vi "ni_monoDrive.vi"() -> ()   [LabVIEW 2018]
uses:
  f4205ffc-a547-4453-97f1-55d6d4306e88.vi
panel:
  out "error out":errorcluster
  out "sensor error":errorcluster
  in  "Tab Control":enum32{"Vehicle", "Environment"}(tab)
  out "Sensor Config":string
  in  "Sensor Configuration":path
  in  "Simulator Configuration":path
  out "Simulator Config":string
  in  "Python Module Path":path
  in  "Steering Angle":dbl(knob) scale=-1.0..1.0
  out "Waveform Chart":dbl(graph)
  out "Speed":dbl(knob) scale=0.0..200.0
  in  "stop":bool
  in  "Throttle":dbl(slide) scale=-1.0..1.0
  out "camera_out 2":picture
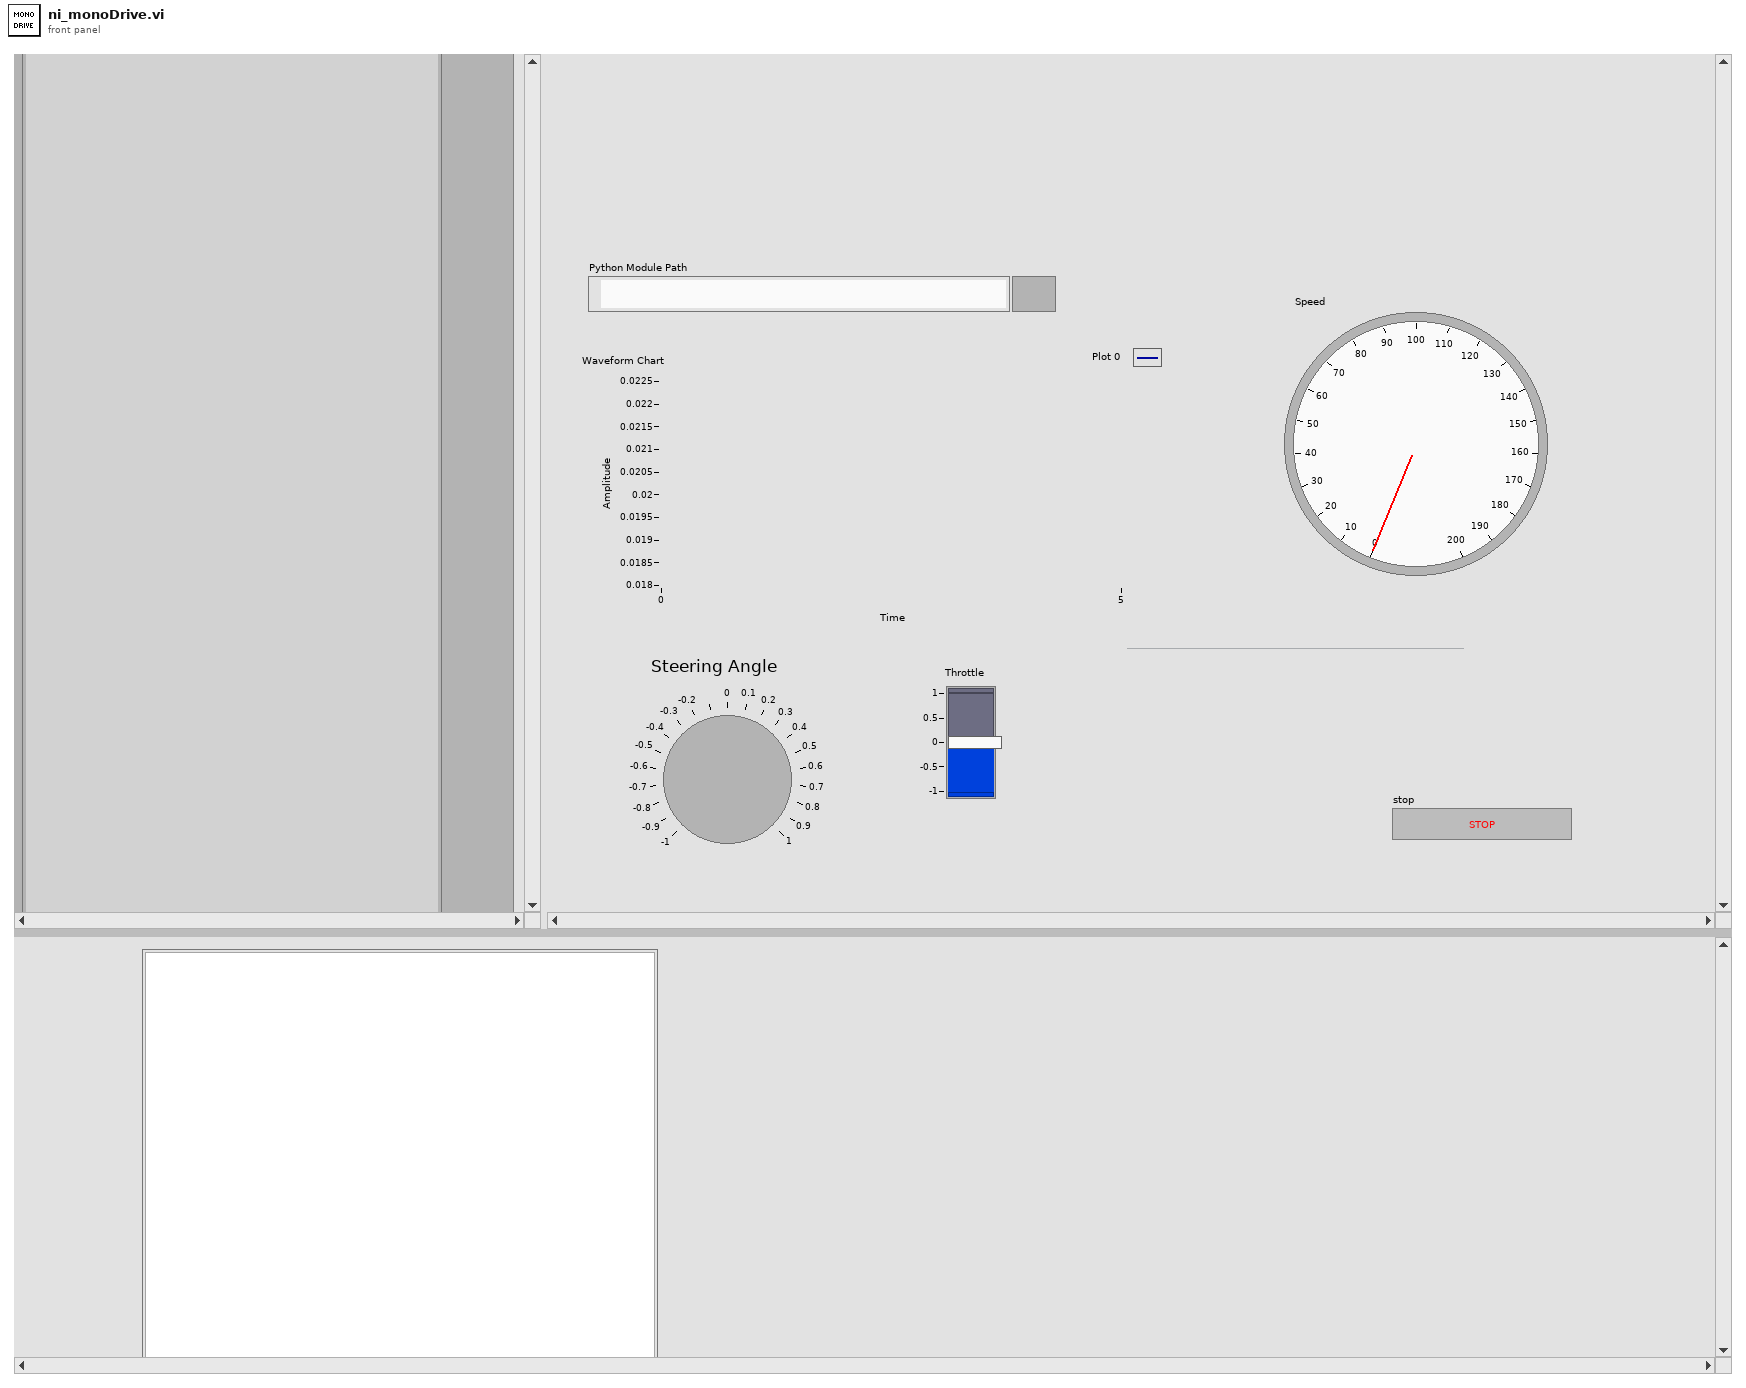
[diagram p1: front panel]
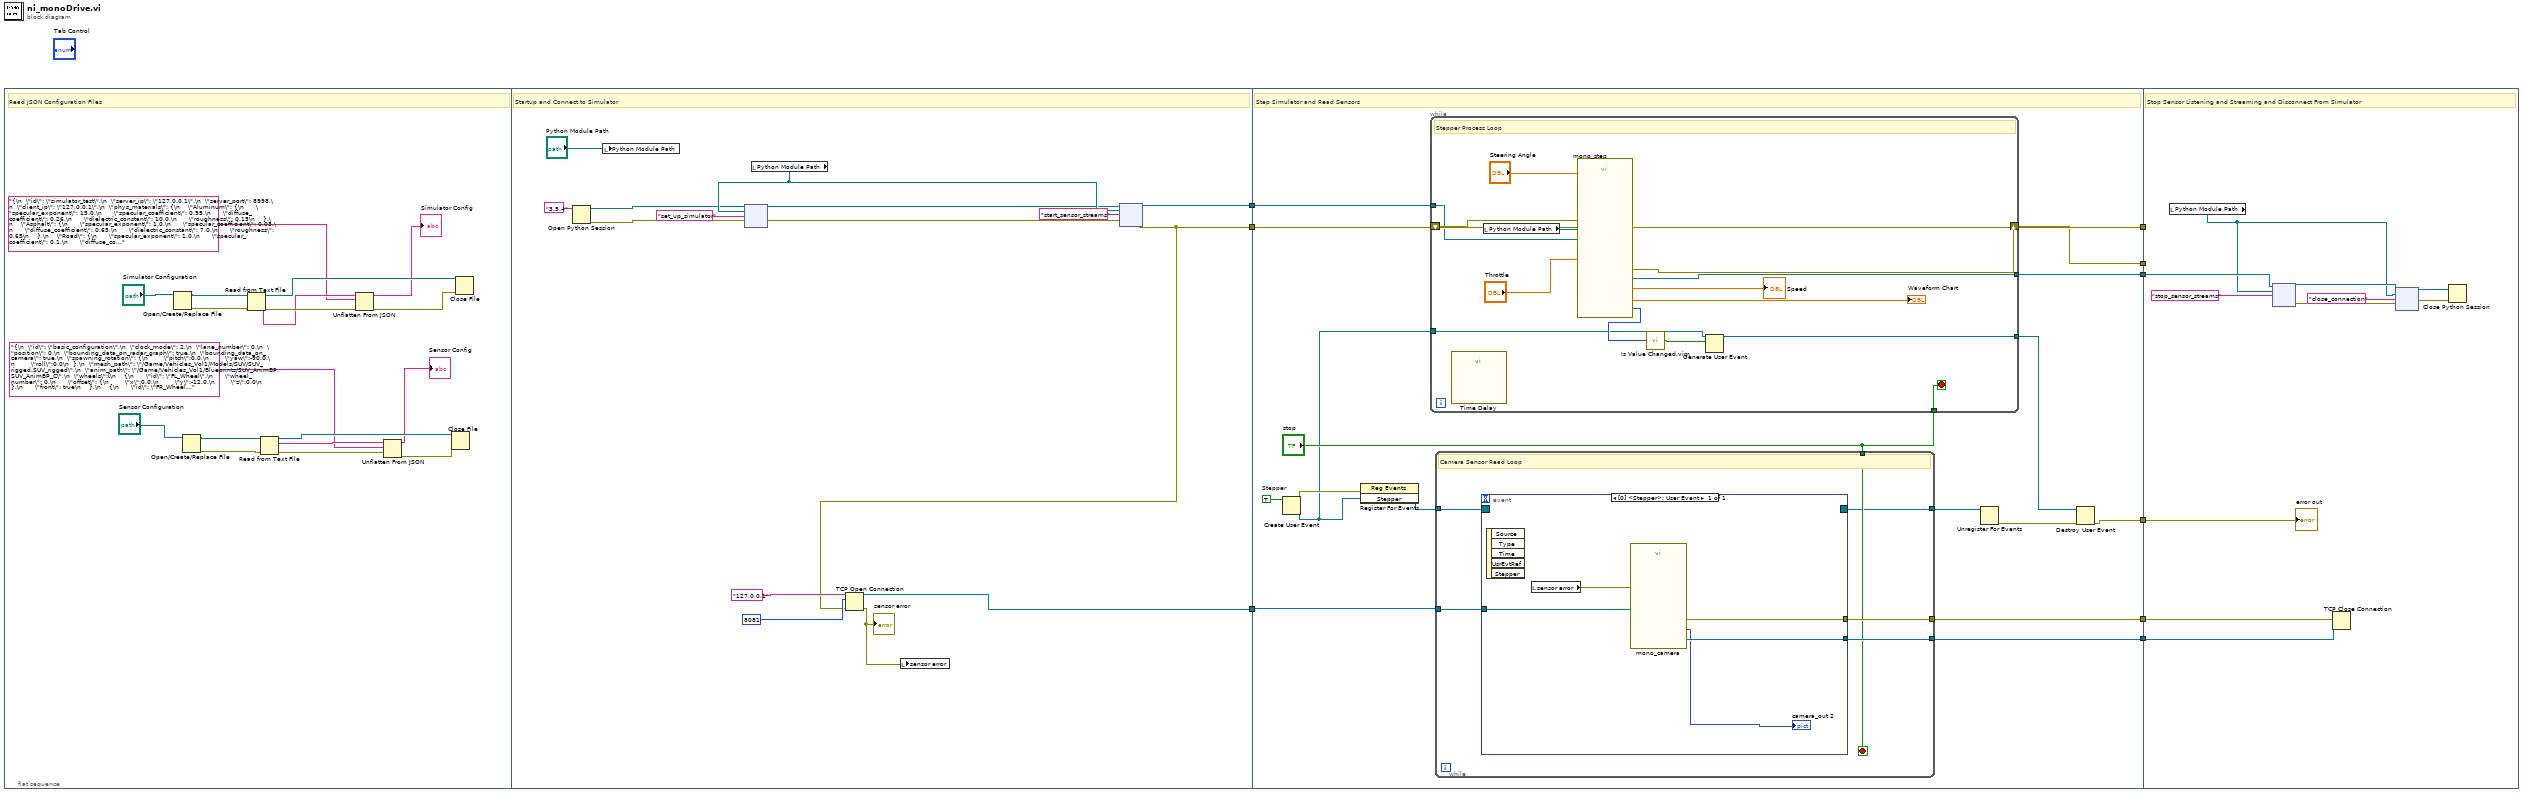
[diagram p0: block diagram]
diagram:
  n1 = flat-sequence {
    tunnel: [w28] -> w9
    tunnel: [w30] -> w4
    tunnel: [w29] -> w3
    tunnel: w9 -> [w58]
    tunnel: [w58] -> w8
    tunnel: [w57] -> w7
    tunnel: [w56] -> w6
    tunnel: [w55] -> w5
    tunnel: w4 -> [w54]
    tunnel: w3 -> [w53]
    tunnel: [w52] -> w2
    tunnel: [w47] -> w1
    tunnel: w8 -> [_]
    tunnel: w7 -> [_]
    tunnel: w6 -> [w88]
    tunnel: w5 -> [w87]
    tunnel: w2 -> [w86]
    tunnel: w1 -> [w84]
    frame #0 {
      # "Read JSON Configuration Files"
      n2 = Open/Create/Replace File(file path (use dialog)="Simulator Configuration") -> (refnum out=w17:refnum<file>, error out=w15:errorcluster)  [unwired: 5 in, 1 out]
      n3 = Open/Create/Replace File(file path (use dialog)="Sensor Configuration") -> (refnum out=w26:refnum<file>, error out=w24:errorcluster)  [unwired: 5 in, 1 out]
      n4 = Read from Text File(file (use dialog)=w17, error in=w15) -> (refnum out=w16:refnum<file>, text=w12:string, error out=w14:errorcluster)  [unwired: 2 in, 1 out]
      n5 = Read from Text File(file (use dialog)=w26, error in=w24) -> (refnum out=w25:refnum<file>, text=w21:string, error out=w23:errorcluster)  [unwired: 2 in, 1 out]
      n6 = Unflatten From JSON(JSON string=w12, type and defaults="{\n  \"id\": \"simulator_test\",\n  \"server_ip\": \"127.0.0.1\",\n  \"server_port\": 8998,\n  \"client_ip\": \"127.0.0.1\",\n  \"phys_materials\": {\n    \"Aluminum\": {\n      \"specular_exponent\": 15.0,\n      \"specular_coefficient\": 0.95,\n      \"diffuse_coefficient\": 0.26,\n      \"dielectric_constant\": 10.0,\n      \"roughness\": 0.15\n    },\n    \"Asphalt\": {\n      \"specular_exponent\": 1.0,\n      \"specular_coefficient\": 0.03,\n      \"diffuse_coefficient\": 0.65,\n      \"dielectric_constant\": 7.0,\n      \"roughness\": 0.65\n    },\n    \"Road\": {\n      \"specular_exponent\": 1.0,\n      \"specular_coefficient\": 0.1,\n      \"diffuse_coefficient\": 0.65,\n      \"dielectric_constant\": 7.0,\n      \"roughness\": 0.65\n    },\n    \"Concrete\": {\n      \"specular_exponent\": 0.0,\n      \"specular_coefficient\": 0.1,\n      \"diffuse_coefficient\": 0.65,\n      \"dielectric_constant\": 7.0,\n      \"roughness\": 0.0\n    },\n    \"Glass\": {\n      \"specular_exponent\": 80.0,\n      \"specular_coefficient\": 0.80,\n      \"diffuse_coefficient\": 0.15,\n      \"dielectric_constant\": 4.0,\n      \"roughness\": 0.10\n    },\n    \"LandScape\": {\n      \"specular_exponent\": 10.0,\n      \"specular_coefficient\": 0.50,\n      \"diffuse_coefficient\": 0.50,\n      \"dielectric_constant\": 10.0,\n      \"roughness\": 0.60\n    },\n    \"Plastic\": {\n      \"specular_exponent\": 25.0,\n      \"specular_coefficient\": 0.40,\n      \"diffuse_coefficient\": 0.60,\n      \"dielectric_constant\": 2.8,\n      \"roughness\": 0.09\n    },\n    \"Steel\": {\n      \"specular_exponent\": 26.0,\n      \"specular_coefficient\": 1.0,\n      \"diffuse_coefficient\": 0.33,\n      \"dielectric_constant\": 0.0,\n      \"roughness\": 0.23\n    },\n    \"Tree\": {\n      \"specular_exponent\": 10.0,\n      \"specular_coefficient\": 0.05,\n      \"diffuse_coefficient\": 0.97,\n      \"dielectric_constant\": 10.0,\n      \"roughness\": 0.60\n    },\n    \"Wheel\": {\n      \"specular_exponent\": 92.0,\n      \"specular_coefficient\": 0.95,\n      \"diffuse_coefficient\": 0.06,\n      \"dielectric_constant\": 10.0,\n      \"roughness\": 0.15\n    },\n    \"Tire\": {\n      \"specular_exponent\": 25.0,\n      \"specular_coefficient\": 0.40,\n      \"diffuse_coefficient\": 0.60,\n      \"dielectric_constant\": 2.8,\n      \"roughness\": 0.15\n    }\n  },\n  \"traffic_configuration\": {\n    \"max_vehicles\": 40,\n    \"spawn_rate\": 0.25\n  },\n  \"client_settings\": {\n    \"map\": {\n      \"gis_anchor\": { \"x\": 0, \"y\": 0, \"z\": 0},\n      \"point_delta\": 100.0\n    },\n    \"gui\":{\n      \"fps\": 1.0\n    },\n    \"logger\": {\n      \"sensor\": \"debug\",\n      \"network\": \"debug\",\n      \"control\": \"debug\",\n      \"scenario\": \"debug\",\n      \"simulator\": \"debug\",\n      \"vehicle\": \"debug\"\n    }\n  }\n}\n" ("function name"), error in (no error)=w14) -> (value=→"Simulator Config":string, error out=w13:errorcluster)  [unwired: 4 in]
      n7 = Unflatten From JSON(JSON string=w21, type and defaults="{\n  \"id\": \"basic_configuration\",\n  \"clock_mode\": 2,\n  \"lane_number\": 0,\n  \"position\": 0,\n  \"bounding_data_on_radar_graph\": true,\n  \"bounding_data_on_camera\": true,\n  \"spawning_rotation\": {\n        \"pitch\":0.0,\n        \"yaw\":-90.0,\n        \"roll\":0.0\n  },\n  \"mesh_path\": \"/Game/Vehicles_Vol1/Models/SUV/SUV_rigged.SUV_rigged\",\n  \"anim_path\": \"/Game/Vehicles_Vol1/Blueprints/SUV_AnimBP.SUV_AnimBP_C\",\n  \"wheels\":[\n    {\n      \"id\": \"FL_Wheel\",\n      \"wheel_number\": 0,\n      \"offset\": {\n        \"x\":0.0,\n        \"y\":-12.0,\n        \"z\":0.0\n      },\n      \"front\": true\n    },\n    {\n      \"id\": \"FR_Wheel\",\n      \"wheel_number\": 1,\n      \"offset\": {\n        \"x\":0.0,\n        \"y\":12.0,\n        \"z\":0.0\n      },\n      \"front\": true\n    },\n    {\n      \"id\": \"BL_Wheel\",\n      \"wheel_number\": 2,\n      \"offset\": {\n        \"x\":0.0,\n        \"y\":-12.0,\n        \"z\":0.0\n      },\n      \"front\": false\n    },\n    {\n      \"id\": \"BR_Wheel\",\n      \"wheel_number\": 3,\n      \"offset\": {\n        \"x\":0.0,\n        \"y\":12.0,\n        \"z\":0.0\n      },\n      \"front\": false\n    }\n  ],\n  \"sensors\": [\n      {\n      \"type\": \"Lidar\",\n      \"id\": \"0\",\n      \"packet_size\": 1472,\n      \"listen_port\": 8089,\n      \"display_process\": true,\n      \"sensor_process\": true,\n      \"synchronized_display\": true,\n      \"location\": {\n        \"x\":-75.0,\n        \"y\":-25.0,\n        \"z\":350.0\n      },\n      \"rotation\": {\n        \"pitch\":0.0,\n        \"yaw\":0.0,\n        \"roll\":0.0\n      },\n      \"max_distance\": 8000.0,\n      \"vertical_fov_angle\": 30.0,\n      \"horizontal_resolution\": 0.4,\n      \"fps\": 1.0,\n      \"n_lasers\": 32,\n      \"reset_angle\": 0.0\n    },\n    {\n      \"type\": \"Radar\",\n      \"id\": \"2\",\n      \"packet_size\": 64000,\n      \"listen_port\": 8088,\n      \"display_process\": true,\n      \"sensor_process\": true,\n      \"synchronized_display\": true,\n      \"location\": {\n        \"x\": 250.0,\n        \"y\": 0.0,\n        \"z\": 50.0\n      },\n      \"rotation\": {\n        \"pitch\": 0.0,\n        \"yaw\": 0.0,\n        \"roll\": 0.0\n      },\n      \"num_samples_per_sweep\": 1100,\n      \"fs\": 150000000,\n      \"fc\": 77000000000.0,\n      \"num_sweeps\": 64,\n      \"range_max\": 150.0,\n      \"sweep_num_for_range_max\": 5.5,\n      \"range_resolution\": 1.0,\n      \"max_velocity\": 100.0,\n      \"max_targets\": 100,\n      \"fps\": 1.0,\n      \"elements\": 8,\n      \"transmitter\": {\n        \"peak_power\": 5.0,\n        \"aperture\": 0.000859,\n        \"gain\": 13.5\n      },\n      \"receiver\": {\n        \"aperture\": 0.000798,\n        \"nf\": 10.0,\n        \"noise_temp\": 290.0,\n        \"nb\": 74000000.0,\n        \"gain\": 20.0,\n        \"kb\": 0.00059641065\n      },\n      \"sbr\": {\n        \"minimum_radar_distance\": 5.0,\n        \"long_range_scan_distance\": 150.0,\n        \"short_range_scan_distance\": 60.0,\n        \"num_scans_azimuth\": 20.0,\n        \"long_range_fov\": 20.0,\n        \"short_range_fov\": 90.0,\n        \"num_scans_elevation\": 10.0,\n        \"elevation_fov\": 5.0,\n        \"max_raycast_hits\": 1\n      }\n    },\n    {\n      \"type\":\"Camera\",\n      \"id\": \"0\",\n      \"packet_size\": 1472,\n      \"listen_port\": 8081,\n      \"display_process\": true,\n      \"sensor_process\": true,\n      \"synchronized_display\": true,\n      \"location\": {\n        \"x\":-600.0,\n        \"y\":0.0,\n        \"z\":400.0\n      },\n      \"rotation\": {\n        \"pitch\":-20.0,\n        \"yaw\":0.0,\n        \"roll\":0.0\n      },\n      \"max_distance\": 50000.0,\n      \"horizontal_fov_angle\": 70.0,\n      \"fps\": 1.0,\n      \"stream_dimensions\": {\n        \"x\":512.0,\n        \"y\":512.0\n      },\n      \"semantic_processing\": false,\n      \"hdmi_streaming\": false\n    },\n    {\n      \"type\": \"BoundingBox\",\n      \"id\": \"1\",\n      \"packet_size\": 1472,\n      \"listen_port\": 8082,\n      \"display_process\": true,\n      \"sensor_process\": true,\n      \"synchronized_display\": true,\n      \"location\": {\n        \"x\":-75.0,\n        \"y\":-25.0,\n        \"z\":245.0\n      },\n      \"rotation\": {\n        \"pitch\":0.0,\n        \"yaw\":0.0,\n        \"roll\":0.0\n      },\n      \"fps\": 1.0\n    },\n    {\n      \"type\": \"Waypoint\",\n      \"id\": \"4\",\n      \"packet_size\": 1472,\n      \"listen_port\": 8083,\n      \"display_process\": false,\n      \"sensor_process\": true,\n      \"synchronized_display\": true,\n      \"location\": {\n        \"x\": 0.0,\n        \"y\": 0.0,\n        \"z\": 0.0\n      },\n      \"rotation\": {\n        \"pitch\": 0.0,\n        \"yaw\": 0.0,\n        \"roll\": 0.0\n      },\n      \"fps\": 1.0,\n      \"point_delta\": 100.0,\n      \"total_points\": 100.0\n    },\n    {\n      \"type\": \"GPS\",\n      \"id\": \"0\",\n      \"packet_size\": 1472,\n      \"listen_port\": 8084,\n      \"display_process\": true,\n      \"sensor_process\": true,\n      \"synchronized_display\": true,\n      \"location\": {\n        \"x\": -75.0,\n        \"y\": -25.0,\n        \"z\": 245.0\n      },\n      \"rotation\": {\n        \"pitch\": 0.0,\n        \"yaw\": 0.0,\n        \"roll\": 0.0\n      },\n      \"fps\": 1.0\n    },\n    {\n      \"type\": \"IMU\",\n      \"id\": \"0\",\n      \"packet_size\": 1472,\n      \"listen_port\": 8085,\n      \"display_process\": true,\n      \"sensor_process\": true,\n      \"synchronized_display\": true,\n      \"location\": {\n        \"x\":-75.0,\n        \"y\":-25.0,\n        \"z\":245.0\n      },\n      \"rotation\": {\n        \"pitch\":0.0,\n        \"yaw\":0.0,\n        \"roll\":0.0\n      },\n      \"fps\": 1.0\n    },\n    {\n      \"type\": \"RPM\",\n      \"id\": \"0\",\n      \"packet_size\": 1472,\n      \"listen_port\": 8086,\n      \"display_process\": false,\n      \"sensor_process\": false,\n      \"location\": {\n        \"x\": 0,\n        \"y\": 0,\n        \"z\": 0\n      },\n      \"rotation\": {\n        \"pitch\": 0,\n        \"yaw\": 0,\n        \"roll\": 0\n      },\n      \"fps\": 1.0,\n      \"wheel_number\": 0\n    }\n  ]\n}" ("function name"), error in (no error)=w23) -> (value=→"Sensor Config":string, error out=w22:errorcluster)  [unwired: 4 in]
      n8 = Close File(refnum=w25, error in=w22) -> ()  [unwired: 2 out]
      n9 = Close File(refnum=w16, error in=w13) -> ()  [unwired: 2 out]
    }
    frame #1 {
      # "Startup and Connect to Simulator"
      n10 = Open Python Session(python version="3.5.4" ("Python version")) -> (session out=w37:refnum<k35>, error out=w38:errorcluster)  [unwired: 2 in]
      n11 = local write "Python Module Path"("Python Module Path") -> ()
      n12 = local read "Python Module Path"() -> (w41:path)
      n13 = node(w37, w41, "set_up_simulator" ("function name"), w38) -> (w39:refnum<k35>, w40:errorcluster)  [unwired: 2 in, 2 out]
      n14 = node(w39, w41, "start_sensor_streams" ("function name"), w40) -> (w29:refnum<k35>, w28:errorcluster)  [unwired: 2 in, 2 out]
      n15 = TCP Open Connection(address="127.0.0.1", remote port or service name=u16 8081, error in (no error)=w28) -> (connection ID=w30:refnum<k5>, error out=w31:errorcluster)  [unwired: 2 in]
      "sensor error" <- w31
      n16 = local write "sensor error"(w31) -> ()
    }
    frame #2 {
      w45 = TRUE  # Stepper
      # "Step Simulator and Read Sensors"
      n17 = Create User Event ("Step Event\nStep Event")(user event datatype=w45) -> (user event=w43:refnum<user-event>, error out=w46:errorcluster)  [unwired: 1 in]
      n18 = register-events(error in=w46, w43) -> (reference out=w50:refnum<event-registration>)  [unwired: 1 in, 1 out]
      n19 = while {
        shift-right: [w74] -> w57
        shift-left: _ -> [w83]
        tunnel: w53 -> [w77]
        tunnel: [w76] -> w52
        tunnel: "stop" -> [w75]
        tunnel: [w72] -> w44
        tunnel: w43 -> [w70]
        stop <- w75 stop-if-true
        # "Stepper Process Loop"
        n20 = call "Time Delay"() -> ()  [unwired: 11 in, 1 out]
        n21 = local read "Python Module Path"() -> (w79:path)
        n22 = call "mono_step.vi"("Steering Wheel Angle"="Steering Angle", "error_in"=w83, "Throttle"="Throttle", "Python Module Path"=w79, "Refnum in"=w77) -> ("error_out"=w74:errorcluster, "Waveform Chart"=→"Waveform Chart":dbl, "Speed"=→"Speed":dbl, "Refnum out"=w76:refnum<k35>, "return value"=w73:i32[])  [unwired: 2 in]
        n23 = call "Is Value Changed.vim"("value"=w73) -> ("changed or first call?"=w71:bool)
        n24 = Generate User Event(user event=w70, event data cluster=w71) -> (user event out=w72:refnum<user-event>)  [unwired: 2 in, 1 out]
      }
      n25 = while {
        tunnel: [w64] -> w56
        tunnel: [w63] -> w55
        tunnel: "stop" -> [w62]
        tunnel: w54 -> [w61]
        tunnel: w50 -> [w60]
        tunnel: [w59] -> w49
        stop <- w62 stop-if-true
        # "Camera Sensor Read Loop"
        n26 = event shown="[0] <Stepper>: User Event" {
          selector: w60 -> [_]
          dyn-events: [_] -> w59
          timeout: _ -> [_]
          tunnel: [w69] -> w64
          tunnel: [w68] -> w63
          tunnel: w61 -> [w66]
          event User Event {
            n27 = event-data() -> ()  [unwired: 1 in, 5 out]
            n28 = local read "sensor error"() -> (w67:errorcluster)
            n29 = call "mono_camera.vi"("error in"=w67, "tcp_in"=w66) -> ("error out"=w69:errorcluster, "camera_out"=→"camera_out 2":picture, "tcp_out"=w68:refnum<k5>)  [unwired: 7 in]
          }
        }
      }
      n30 = Unregister For Events(event registration refnum=w49) -> (error out=w48:errorcluster)  [unwired: 1 in]
      n31 = Destroy User Event(user event=w44, error in=w48) -> (error out=w47:errorcluster)
    }
    frame #3 {
      # "Stop Sensor Listening and Streaming and Disconnect From Simulator"
      n32 = local read "Python Module Path"() -> (w85:path)
      n33 = node(w86, w85, "stop_sensor_streams" ("function name")) -> (w94:refnum<k35>, w93:errorcluster)  [unwired: 3 in, 2 out]
      n34 = TCP Close Connection(connection ID=w87, error in (no error)=w88) -> ()  [unwired: 1 in, 2 out]
      n35 = node(w94, w85, "close_connection" ("function name"), w93) -> (w92:refnum<k35>, w91:errorcluster)  [unwired: 2 in, 2 out]
      n36 = Close Python Session(session in=w92, error in=w91) -> ()  [unwired: 1 out]
      "error out" <- w84
    }
  }
